vi "Initialize.vi"(7 "error in":errorcluster, 10 "ChassisType":T1) -> (0 "error out":errorcluster, 3 "Chassis Cfg":refnum<class "ChassisCfg.lvclass">)   [LabVIEW 2018, in "Configuration Grandmaster.lvlib" / "ChassisCfg.lvclass"]
uses:
  ChassisCfg.lvclass
  Common/Controls/Chassis Type.ctl
  Common/Controls/LS Lock Sizes.ctl
  ChassisCfg.lvclass/ChassisCfg.ctl
  Class Timing Group/TimingGrp.lvclass
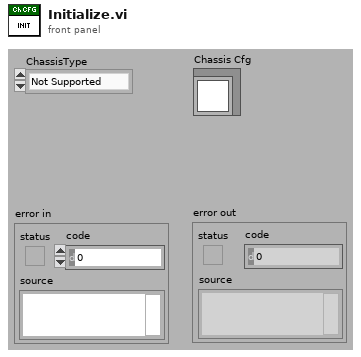
[diagram p1: front panel]
types:
  T1 = typedef "Chassis Type.ctl" = enum16{"Not Supported", "C Series 1-Slot", "C Series 4-Slot", "C Series 8-Slot", "PXI 8-Slot", "PXIe 18-Slot"}
  T2 = typedef "LS Lock Sizes.ctl" = enum16{"No", "250ms", "500ms", "1s"}
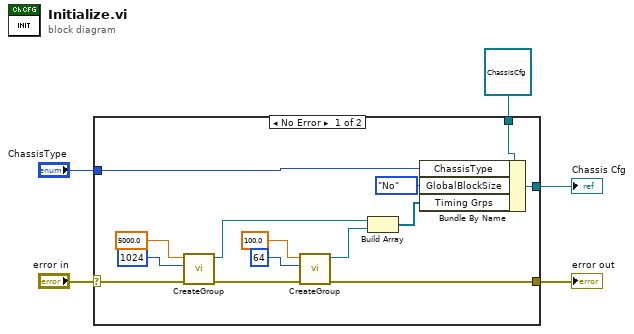
[diagram p0: block diagram]
diagram:
  n1 = case shown="No Error" "error in" {
    selector: "error in" -> [w12 w21]
    tunnel: [w19 w20] -> w2
    tunnel: [w13 w21] -> w5
    tunnel: refnum<class "ChassisCfg.lvclass"> refnum ("Chassis Cfg") -> [w11 w20]
    tunnel: "ChassisType" -> [w6 _]
    frame No Error {
      n2 = call "CreateGroup.vi"("error in"=w12, "ReadBlk"=1024, "Rate"=5000.0) -> ("error out"=w16:errorcluster, "Timing Group"=w9:refnum<class "TimingGrp.lvclass">)  [unwired: 7 in]
      n3 = call "CreateGroup.vi"("error in"=w16, "ReadBlk"=64, "Rate"=100.0) -> ("error out"=w13:errorcluster, "Timing Group"=w8:refnum<class "TimingGrp.lvclass">)  [unwired: 7 in]
      n4 = Build Array(w9, w8) -> (w7:refnum<class "TimingGrp.lvclass">[])
      n5 = Bundle By Name(cluster=w11, "ChassisType"=w6, "GlobalBlockSize"=LS_Lock_Sizes."No", "Timing Grps"=w7) -> (w19:refnum<class "ChassisCfg.lvclass">)
    }
    frame Error {
    }
  }
  "Chassis Cfg" <- w2
  "error out" <- w5
